vi "Example Callback - PMConcentration Callback.vi"(4 "PMConcentration":refnum<user-event>, 5 "Event Data":T1, 6 "Control Ref":refnum<k24>, 7 "Event Common Data":T2) -> ()   [LabVIEW 2013]
uses:
  C:/tf/play/labview/Tinkerforge.dll
  Tinkerforge.dll
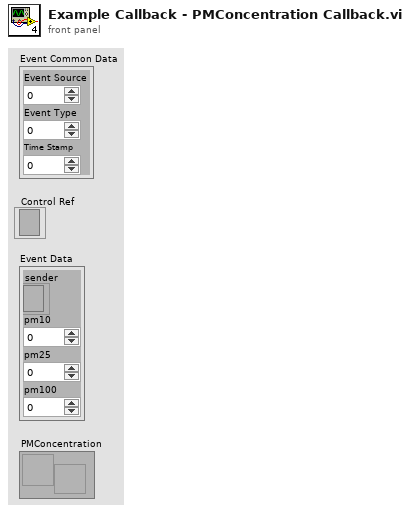
[diagram p1: front panel]
types:
  T1 = cluster{"sender":refnum<k24>, "pm10":i32, "pm25":i32, "pm100":i32}
  T2 = cluster{"Event Source":i32, "Event Type":u32, "Time Stamp":u32}
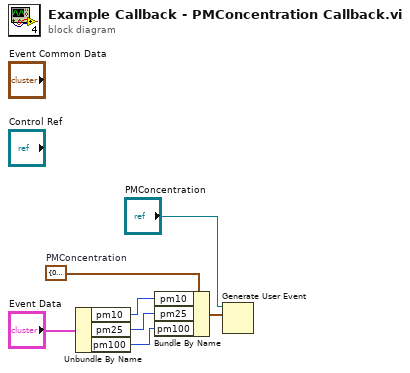
[diagram p0: block diagram]
diagram:
  w7 = cluster{"pm10":i32, "pm25":i32, "pm100":i32} {"pm10"=0, "pm25"=0, "pm100"=0}  # PMConcentration
  n1 = Unbundle By Name("Event Data") -> ("pm10"=w5:i32, "pm25"=w4:i32, "pm100"=w3:i32)
  n2 = Bundle By Name(cluster=w7, "pm10"=w5, "pm25"=w4, "pm100"=w3) -> (w2:cluster{"pm10":i32, "pm25":i32, "pm100":i32})
  n3 = Generate User Event(user event="PMConcentration", event data cluster=w2) -> ()  [unwired: 2 in, 2 out]
